vi "ToSend.vi"(9 "velocity":sgl, 10 "leanAngel":sgl, 11 "setpoint":sgl) -> (3 "data2nRF24":u8[](array[numeric]))   [LabVIEW 2016]
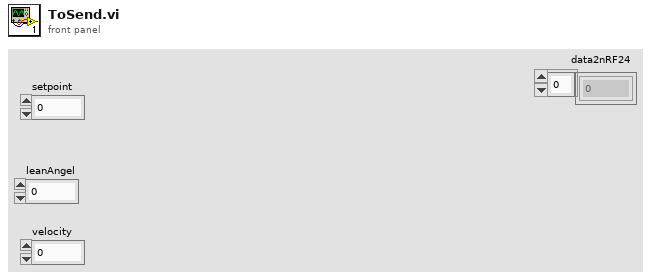
[diagram p1: front panel]
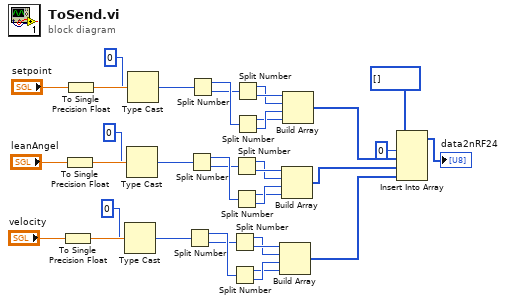
[diagram p0: block diagram]
diagram:
  n1 = To Single Precision Float(number="velocity") -> (single precision float=w15:sgl)
  n2 = To Single Precision Float(number="leanAngel") -> (single precision float=w25:sgl)
  n3 = To Single Precision Float(number="setpoint") -> (single precision float=w35:sgl)
  n4 = Type Cast(type=u32 0, x=w15) -> (*(type *) &x=w13:u32)
  n5 = Type Cast(type=u32 0, x=w25) -> (*(type *) &x=w23:u32)
  n6 = Type Cast(type=u32 0, x=w35) -> (*(type *) &x=w33:u32)
  n7 = Split Number(x=w13) -> (hi(x)=w12:u16, lo(x)=w11:u16)
  n8 = Split Number(x=w23) -> (hi(x)=w22:u16, lo(x)=w21:u16)
  n9 = Split Number(x=w33) -> (hi(x)=w32:u16, lo(x)=w31:u16)
  n10 = Split Number(x=w11) -> (hi(x)=w9:u8, lo(x)=w10:u8)
  n11 = Split Number(x=w12) -> (hi(x)=w7:u8, lo(x)=w8:u8)
  n12 = Split Number(x=w21) -> (hi(x)=w19:u8, lo(x)=w20:u8)
  n13 = Split Number(x=w22) -> (hi(x)=w17:u8, lo(x)=w18:u8)
  n14 = Split Number(x=w31) -> (hi(x)=w29:u8, lo(x)=w30:u8)
  n15 = Split Number(x=w32) -> (hi(x)=w27:u8, lo(x)=w28:u8)
  n16 = Build Array(w10, w9, w8, w7) -> (w4:u8[])
  n17 = Build Array(w20, w19, w18, w17) -> (w5:u8[])
  n18 = Build Array(w30, w29, w28, w27) -> (w6:u8[])
  n19 = Insert Into Array(array=u8[] [], index=0, new element #1=w6, new element #2=w5, new element #3=w4) -> (→"data2nRF24":u8[])
